vi "lok0020_case.vi"() -> ()   [LabVIEW 2020]
uses:
  <vilib>/numeric/Random Number (Range) DBL.vi
panel:
  in  "STOP":bool
  out "Boolean 2":bool
  in  "nabij kotel":bool
  out "Numeric 3":dbl
  out "Numeric 2":u32
  in  "Numeric":u32
  in  "Boolean":bool
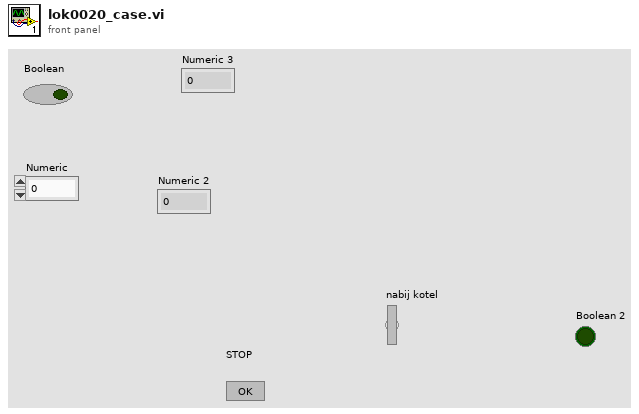
[diagram p1: front panel]
types:
  T1 = enum16{"Timeout", "Power ON", "Power OFF", "Standby", "Init", "Topi", "Netopi"}
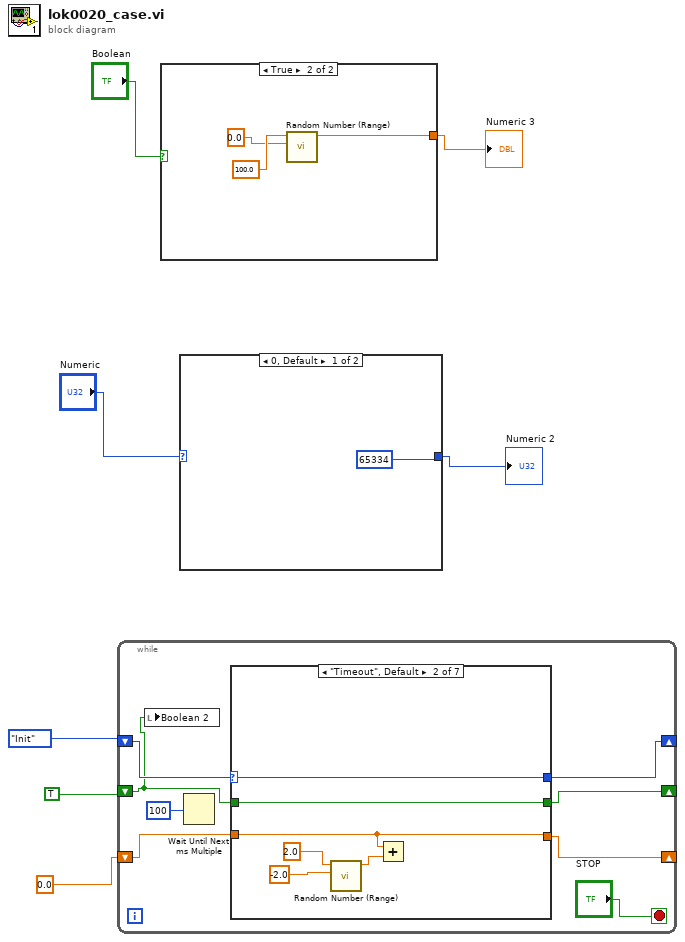
[diagram p0: block diagram]
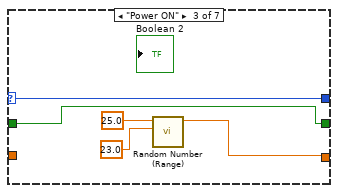
[diagram p3: hidden frame]
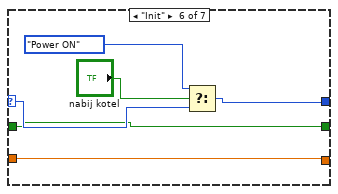
[diagram p6: hidden frame]
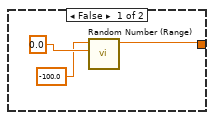
[diagram p9: hidden frame]
diagram:
  n1 = while {
    shift-right: [w14] -> _
    shift-left: T1."Init" -> [w15]
    shift-right: [w12] -> _
    shift-left: 0.0 -> [w13]
    shift-right: [w8] -> _
    shift-left: TRUE -> [w9]
    stop <- "STOP" stop-if-true
    n2 = local write "Boolean 2"(w9) -> ()
    n3 = Wait Until Next ms Multiple(millisecond multiple=100) -> ()  [unwired: 1 out]
    n4 = case shown="\"Timeout\", Default" w15 {
      selector: w15 -> [w18 w24 w29 w32 w35 w41 w44]
      tunnel: [w18 w24 w29 w32 w35 w38 w44] -> w14
      tunnel: [w17 w19 w26 w31 w34 w37 w43] -> w12
      tunnel: w13 -> [w17 w19 _ w31 w34 w37 w43]
      tunnel: w9 -> [w16 w23 w25 w30 w33 w36 w42]
      tunnel: [w16 w23 w25 w30 w33 w36 w42] -> w8
      frame "Netopi" {
      }
      frame "Timeout", Default {
        n5 = call-poly <vilib>:"Random Number (Range).vi"("lower bound (0)"=-2.0, "upper bound (100)"=2.0) -> ("number"=w20:dbl)  [unwired: 9 in]
        n6 = Add(x=w19, y=w20) -> ()  [unwired: 1 out]
      }
      frame "Power ON" {
        n7 = call-poly <vilib>:"Random Number (Range).vi"("lower bound (0)"=23.0, "upper bound (100)"=25.0) -> ("number"=w26:dbl)  [unwired: 9 in]
      }
      frame "Power OFF" {
      }
      frame "Standby" {
      }
      frame "Init" {
        n8 = Select(t=T1."Power ON", s="nabij kotel", f=w41) -> (s? t:f=w38:T1)
      }
      frame "Topi" {
      }
    }
  }
  n9 = case shown="True" "Boolean" {
    tunnel: [w45 w48] -> w4
    frame False {
      n10 = call-poly <vilib>:"Random Number (Range).vi"("lower bound (0)"=0.0, "upper bound (100)"=-100.0) -> ("number"=w45:dbl)  [unwired: 9 in]
    }
    frame True {
      n11 = call-poly <vilib>:"Random Number (Range).vi"("lower bound (0)"=0.0, "upper bound (100)"=100.0) -> ("number"=w48:dbl)  [unwired: 9 in]
    }
  }
  "Numeric 3" <- w4
  n12 = case shown="0, Default" "Numeric" {
    selector: "Numeric" -> [_ w52]
    tunnel: [65334 w52] -> w5
    frame 0, Default {
    }
    frame 1 {
    }
  }
  "Numeric 2" <- w5
